vi "ATA10003-Config.vi"(6 "Frequency(Hz)":dbl=60.0, 7 "Delay Time (s)":dbl=0.5, 8 "error in":errorcluster caption="错误输入（无错误）", 9 "Current(mA)":dbl=500.0, 10 "Voltage(V)":dbl=230.0, 11 "MyIndex":u8) -> (0 "error out":errorcluster, 3 "Result":bool)   [LabVIEW 2015]
uses:
  <vilib>/Instr/_visa.llb/VISA Configure Serial Port (Instr).vi
panel:
  in  "Address(0x01)":u8=1 format="%.0x"
  out "VISA":refnum<visa-resource-name>
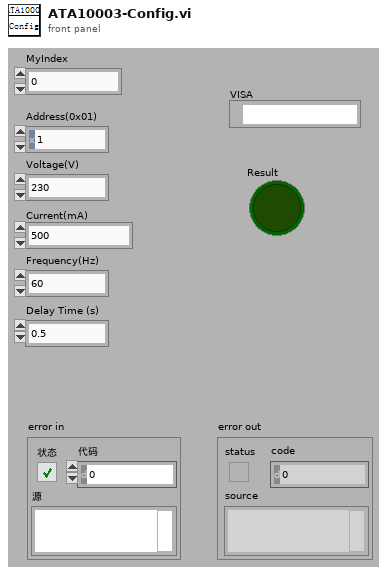
[diagram p1: front panel]
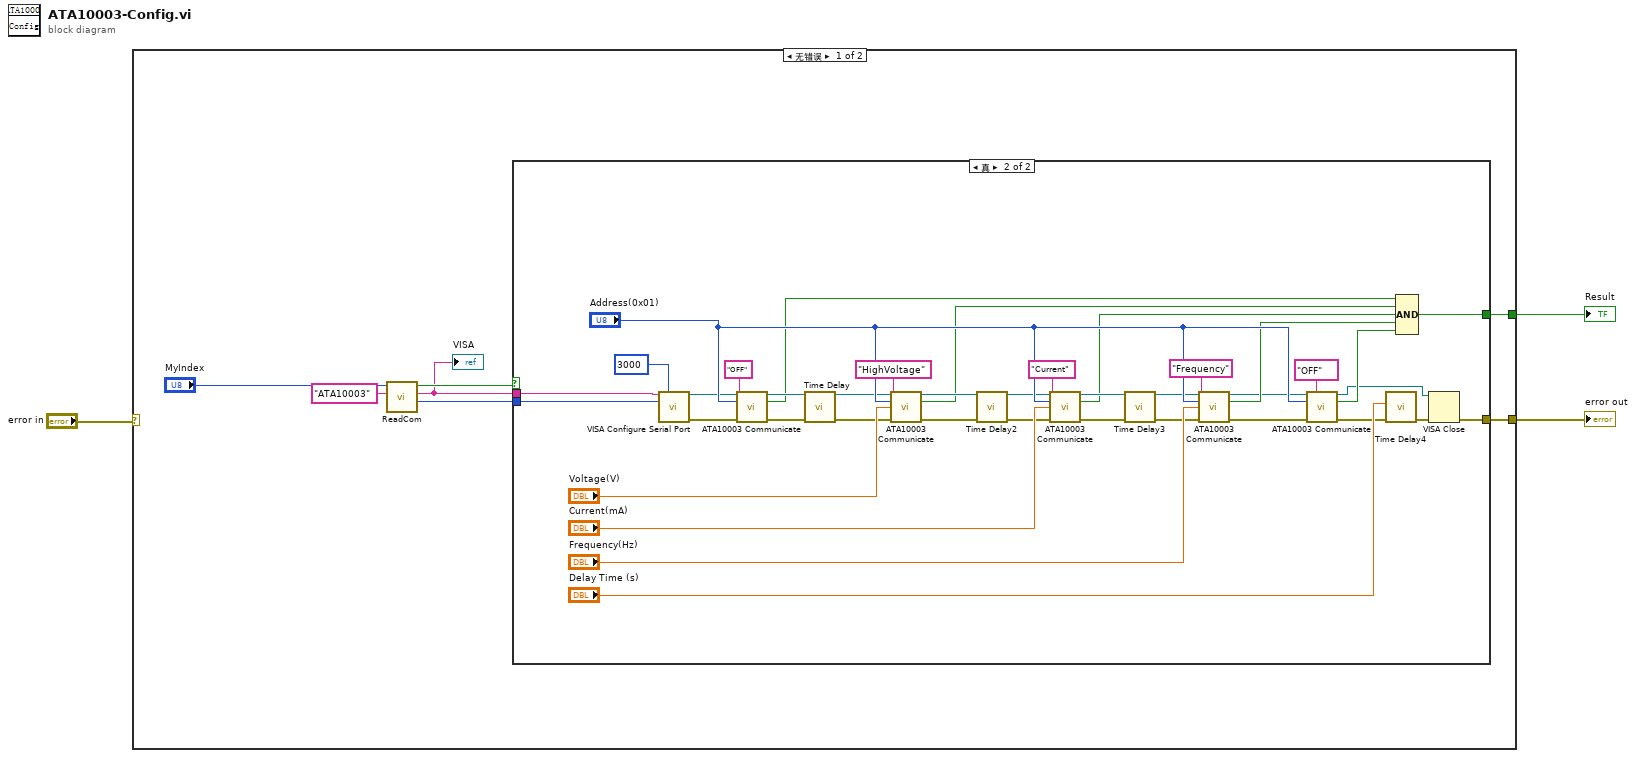
[diagram p0: block diagram]
diagram:
  n1 = case shown="无错误" "error in" {
    selector: "error in" -> [_ w47]
    tunnel: [w10 _] -> w3
    tunnel: [w9 w47] -> w2
    frame No Error {
      n2 = call "ReadCom.vi"("仪器名称"="ATA10003", "MyIndex"="MyIndex") -> ("Baudrate"=w4:i32, "COM"=w5:string, "OK?"=w6:bool)  [unwired: 7 in]
      "VISA" <- w5
      n3 = case shown="真" w6 {
        tunnel: [_ w46] -> w10
        tunnel: [_ w15] -> w9
        tunnel: w5 -> [_ w13]
        tunnel: w4 -> [_ w12]
        frame False {
        }
        frame True {
          n4 = call-poly "VISA Configure Serial Port"("VISA resource name"=w13, "timeout (10sec)"=u32 3000, "baud rate (9600)"=w12) -> ("VISA resource name out"=w30:refnum<visa-resource-name>, "error out"=w33:errorcluster)  [unwired: 11 in]
          n5 = call "ATA10003 Communicate.vi"("VISA Resource In"=w30, "Function_In"="OFF", "Address(0x01)"="Address(0x01)", "error in (no error)"=w33) -> ("VISA Resource Out"=w32:refnum<visa-resource-name>, "OK ?"=w29:bool, "error out"=w31:errorcluster)  [unwired: 7 in, 2 out]
          n6 = call "Time Delay"("error in (no error)"=w31) -> ("error out"=w25:errorcluster)  [unwired: 10 in]
          n7 = call "ATA10003 Communicate.vi"("VISA Resource In"=w32, "Function_In"="HighVoltage", "Address(0x01)"="Address(0x01)", "Value"="Voltage(V)", "error in (no error)"=w25) -> ("VISA Resource Out"=w37:refnum<visa-resource-name>, "OK ?"=w28:bool, "error out"=w24:errorcluster)  [unwired: 6 in, 2 out]
          n8 = call "Time Delay2"("error in (no error)"=w24) -> ("error out"=w23:errorcluster)  [unwired: 10 in]
          n9 = call "ATA10003 Communicate.vi"("VISA Resource In"=w37, "Function_In"="Current", "Address(0x01)"="Address(0x01)", "Value"="Current(mA)", "error in (no error)"=w23) -> ("VISA Resource Out"=w35:refnum<visa-resource-name>, "OK ?"=w27:bool, "error out"=w22:errorcluster)  [unwired: 6 in, 2 out]
          n10 = call "Time Delay3"("error in (no error)"=w22) -> ("error out"=w21:errorcluster)  [unwired: 10 in]
          n11 = call "ATA10003 Communicate.vi"("VISA Resource In"=w35, "Function_In"="Frequency", "Address(0x01)"="Address(0x01)", "Value"="Frequency(Hz)", "error in (no error)"=w21) -> ("VISA Resource Out"=w16:refnum<visa-resource-name>, "OK ?"=w26:bool, "error out"=w19:errorcluster)  [unwired: 6 in, 2 out]
          n12 = call "ATA10003 Communicate.vi"("VISA Resource In"=w16, "Function_In"="OFF", "Address(0x01)"="Address(0x01)", "error in (no error)"=w19) -> ("VISA Resource Out"=w14:refnum<visa-resource-name>, "OK ?"=w17:bool, "error out"=w18:errorcluster)  [unwired: 7 in, 2 out]
          n13 = call "Time Delay4"("error in (no error)"=w18, "Delay Time (s)"="Delay Time (s)") -> ("error out"=w41:errorcluster)  [unwired: 9 in]
          n14 = Compound Arithmetic op=AND(w29, w28, w27, w26, w17) -> (w46:bool)
          n15 = VISA Close(VISA resource name=w14, error in (no error)=w41) -> (error out=w15:errorcluster)
        }
      }
    }
    frame Error {
    }
  }
  "Result" <- w3
  "error out" <- w2
